vi "Destroy.vi"(8 "error in (no error)":errorcluster, 10 "Shared Key":string, 11 "SMO":refnum<class "SMO.lvclass">) -> (0 "error out":errorcluster)   [LabVIEW 2021, in "smo.lvlib" / "SMO.lvclass"]
doc: "Destructor\n\nNote 01: This method is overridable by descendant\nNote 02: When overridden, Call Parent Method is required\n\n---------------------------------------------------------------\nJKI State Machine Objects™\nhttp://jki.net/state-machine-objects/\nCopyright (C) 2005-2015, JKI <info@jki.net>\nALL RIGHTS RESERVED"
uses:
  SMO.lvclass
  SMO.lvclass/SMO.ctl
  Support/Attribute.Owner/Attribute.Owner.lvclass/Attribute.Owner.ctl
  Typedefs/SMOState --Enum.ctl
  Support/Attribute.Owner/Verify Key Match.vi
  Private/GetVariant(Attr).vi
  Private/ReftoDVR--SMO.vi
  Support/Attribute.Owner/Read Shared Key.vi
  Support/Attribute.Owner/Attribute.Owner.lvclass
  Registry/Registry-SMO.lvclass
panel:
  # "For instructions on how to use the JKI State Machine Objects, examples and video tutorials, visit:\nhttp://jki.net/state-machine-objects/\n\nJKI State Machine Objects™\nhttp://jki.net/state-machine-objects/\nCopyright (C) 2005-2015, JKI <info@jki.net>\nALL RIGHTS RESERVED"
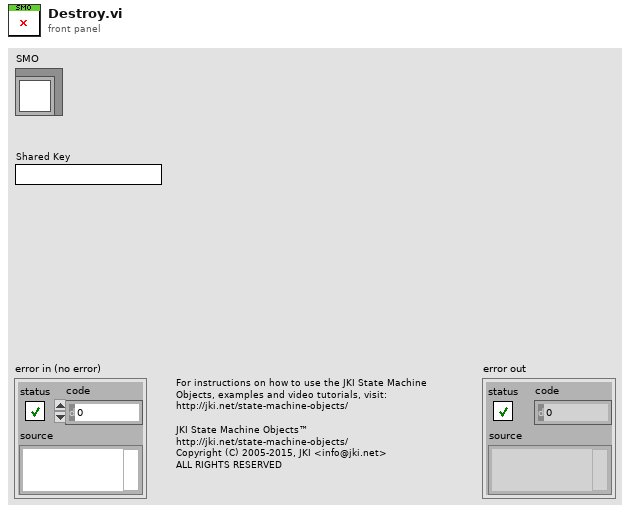
[diagram p1: front panel]
types:
  T1 = typedef "smo.lvlib/SMO.lvclass/SMOState --Enum.ctl" = enum16{"unknown", "Created", "Started", "Stopped"}
  T2 = typedef "smo.lvlib/SMO.lvclass/Public Events.ctl" = cluster{"Error":refnum<user-event>, "State":refnum<user-event>, "Reserve State":refnum<user-event>}
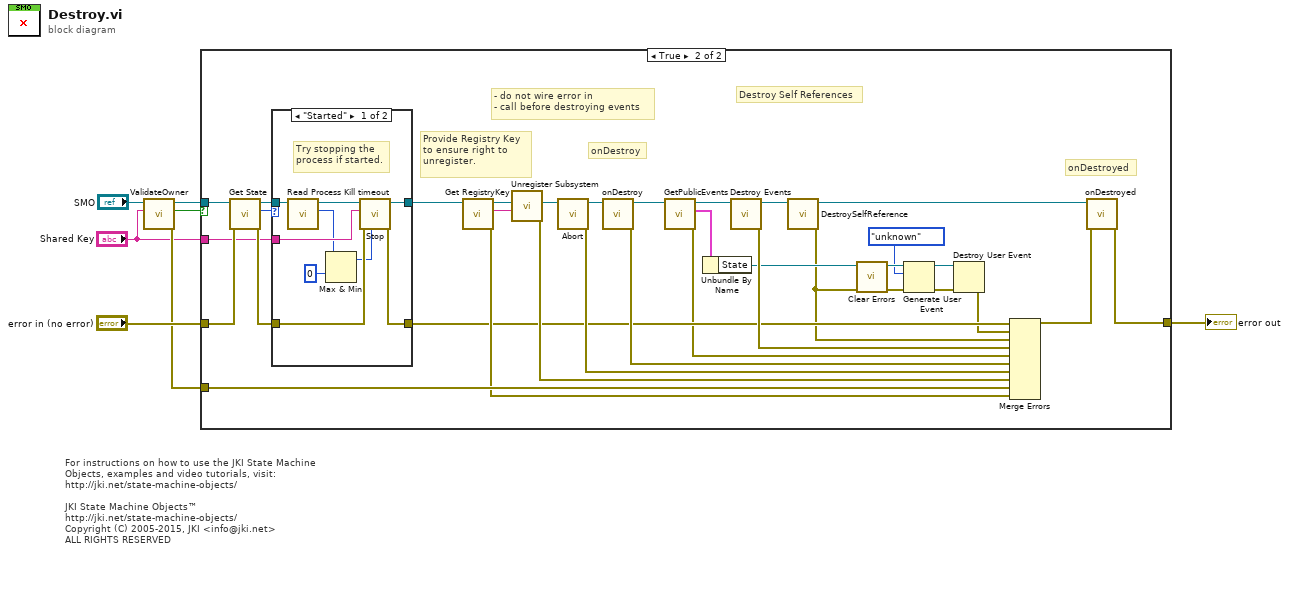
[diagram p0: block diagram]
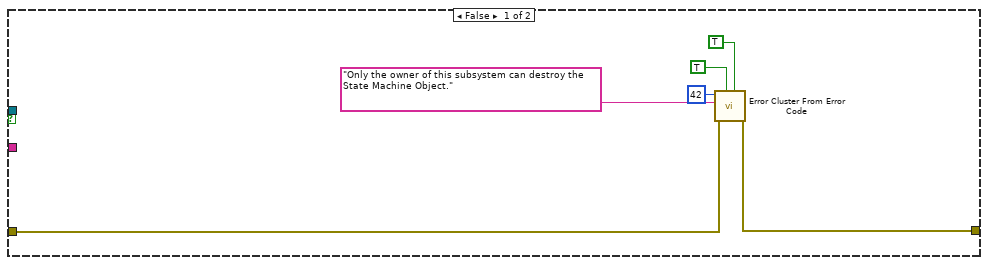
[diagram p2: hidden frame]
diagram:
  # "For instructions on how to use the JKI State Machine Objects, examples and video tutorials, visit:\nhttp://jki.net/state-machine-objects/\n\nJKI State Machine Objects™\nhttp://jki.net/state-machine-objects/\nCopyright (C) 2005-2015, JKI <info@jki.net>\nALL RIGHTS RESERVED"
  n1 = call "ValidateOwner.vi"("Shared Key"="Shared Key", "SMO in"="SMO") -> ("error out"=w3:errorcluster, "key matched"=w2:bool, "SMO out"=w4:refnum<class "SMO.lvclass">)  [unwired: 6 in, 1 out]
  n2 = case shown="True" w2 {
    tunnel: "error in (no error)" -> [w10 w32]
    tunnel: [w9 w42] -> w6
    tunnel: w4 -> [_ w33]
    tunnel: w3 -> [_ w41]
    tunnel: "Shared Key" -> [_ w26]
    frame False {
      n3 = call <vilib>:"Error Cluster From Error Code.vi"("is warning? (False)"=TRUE, "show call chain? (False)"=TRUE, "error in (no error)"=w10, "error message (\"\")"="Only the owner of this subsystem can destroy the State Machine Object." ("error message (\"\")"), "error code (0)"=42) -> ("error out"=w9:errorcluster)  [unwired: 4 in]
    }
    frame True {
      # "Provide Registry Key\nto ensure right to \nunregister."
      # "Destroy Self References"
      # "onDestroy"
      # "onDestroyed"
      # "- do not wire error in\n- call before destroying events"
      n4 = call "Get State.vi"("error in (no error)"=w32, "SMO"=w33) -> ("error out"=w27:errorcluster, "SMO State"=w31:T1, "SMO out"=w30:refnum<class "SMO.lvclass">)  [unwired: 7 in]
      n5 = case shown="\"Started\"" w31 {
        tunnel: w30 -> [w51 w57]
        tunnel: [w54 w57] -> w29
        tunnel: [w52 w56] -> w28
        tunnel: w27 -> [w53 w56]
        tunnel: w26 -> [w55 _]
        frame "Started" {
          # "Try stopping the\nprocess if started."
          n6 = call "Read Process Kill timeout.vi"("SMO in"=w51) -> ("Process Kill timeout (ms)"=w49:i32, "SMO out"=w50:refnum<class "SMO.lvclass">)  [unwired: 9 in]
          n7 = Max & Min(x=w49, y=0) -> (max(x,y)=w48:i32)  [unwired: 1 out]
          n8 = call "Stop.vi"("timeout in ms (-1)"=w48, "error in (no error)"=w53, "Shared Key"=w55, "SMO"=w50) -> ("error out"=w52:errorcluster, "SMO out"=w54:refnum<class "SMO.lvclass">)  [unwired: 6 in]
        }
        frame Default {
        }
      }
      n9 = call "Get RegistryKey.vi"("SMO"=w29) -> ("error out"=w34:errorcluster, "RegistryKey"=w35:string, "SMO out"=w36:refnum<class "SMO.lvclass">)  [unwired: 8 in]
      n10 = call "Unregister Subsystem.vi"("RegistryKey"=w35, "JKI SMO"=w36) -> ("error out"=w44:errorcluster, "JKI SMO out"=w46:refnum<class "SMO.lvclass">)  [unwired: 8 in]
      n11 = call "Abort.vi"("SMO"=w46) -> ("error out"=w45:errorcluster, "SMO out"=w39:refnum<class "SMO.lvclass">)  [unwired: 9 in]
      n12 = call-dynamic "onDestroy.vi"("SMO"=w39) -> ("error out"=w38:errorcluster, "SMO out"=w25:refnum<class "SMO.lvclass">)  [unwired: 9 in]
      n13 = call "GetPublicEvents.vi"("SMO"=w25) -> ("error out"=w23:errorcluster, "Public Events"=w22:T2, "SMO out"=w24:refnum<class "SMO.lvclass">)  [unwired: 8 in]
      n14 = Unbundle By Name(w22) -> ("State"=w21:refnum<user-event>)
      n15 = call "Destroy Events.vi"("SMO"=w24) -> ("error out"=w37:errorcluster, "SMO out"=w14:refnum<class "SMO.lvclass">)  [unwired: 9 in]
      n16 = call-dynamic "DestroySelfReference.vi"("SMO"=w14) -> ("error out"=w18:errorcluster, "SMO out"=w40:refnum<class "SMO.lvclass">)  [unwired: 9 in]
      n17 = call <vilib>:"Clear Errors.vi"("error in (no error)"=w18) -> ("error out"=w19:errorcluster)  [unwired: 5 in, 1 out]
      n18 = Generate User Event(user event=w21, event data cluster=SMOState_--Enum."unknown" ("event data"), error in=w19) -> (user event out=w17:refnum<user-event>, error out=w16:errorcluster)  [unwired: 1 in]
      n19 = Destroy User Event(user event=w17, error in=w16) -> (error out=w15:errorcluster)
      n20 = Merge Errors(w28, w15, w18, w37, w23, w38, w45, w44, w41, w34) -> (w43:errorcluster)
      n21 = call-dynamic "onDestroyed.vi"("error in (no error)"=w43, "SMO"=w40) -> ("error out"=w42:errorcluster)  [unwired: 9 in]
    }
  }
  "error out" <- w6
